vi "SwerveCalculation.vi"(6 "Rot. Point Y":dbl, 7 "Rot. Point X":dbl, 8 "Field Concentric":bool, 9 "Z":dbl(knob) scale=1.0..-1.0, 10 "Y":dbl(slide) scale=1.0..-1.0, 11 "X":dbl(slide) scale=-1.0..1.0) -> ()   [LabVIEW 2016]
uses:
  Robot Global Data.vi
panel:
  in  "Auto Controls":bool
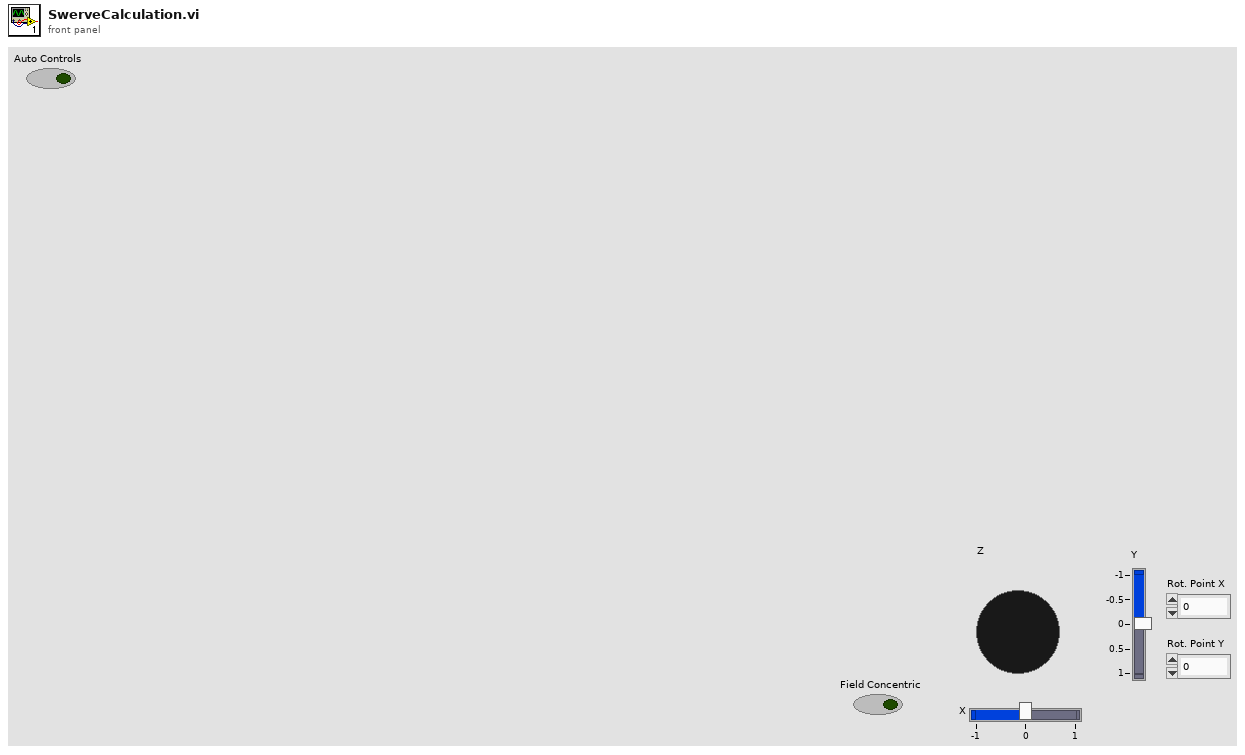
[diagram p1: front panel]
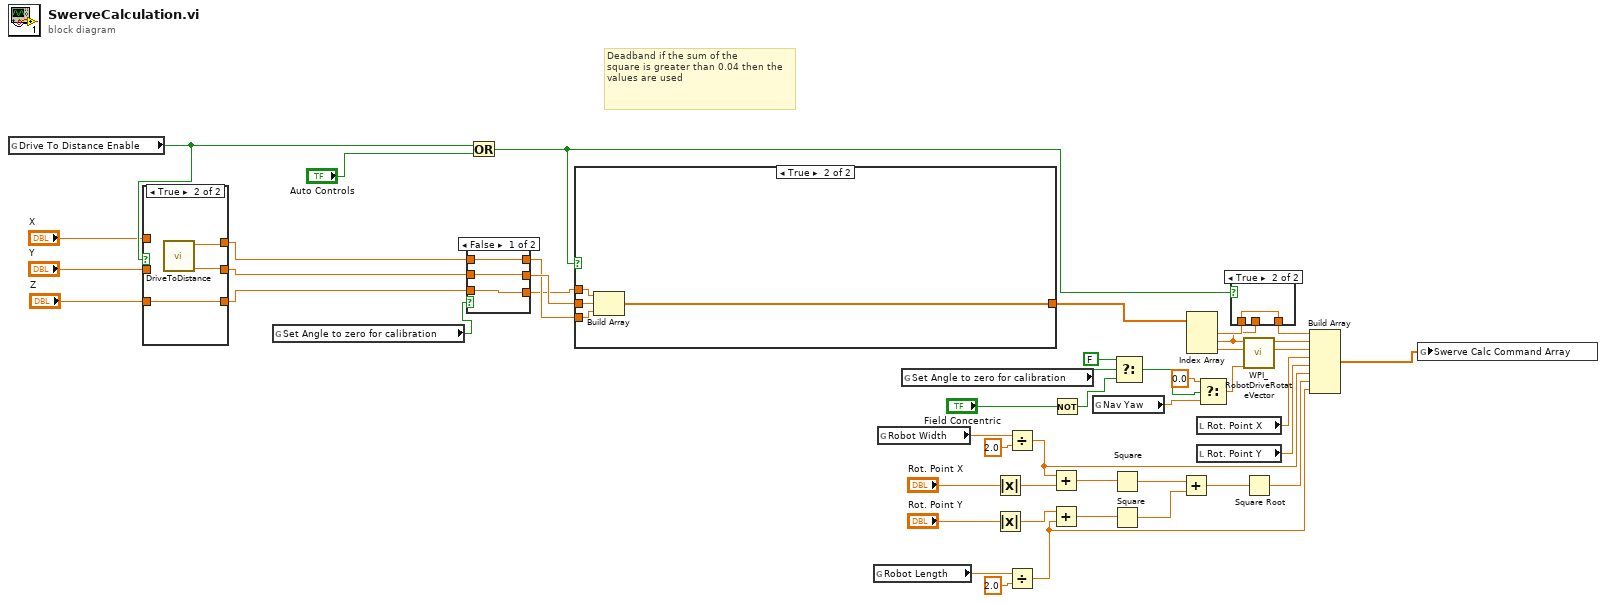
[diagram p0: block diagram]
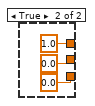
[diagram p3: hidden frame]
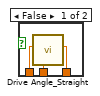
[diagram p4: hidden frame]
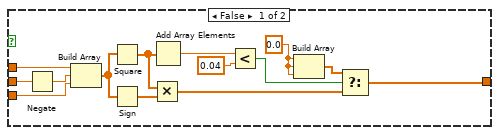
[diagram p5: hidden frame]
diagram:
  # "Deadband if the sum of the \nsquare is greater than 0.04 then the \nvalues are used"
  n1 = global read "Robot Global Data.vi" "Drive To Distance Enable"() -> (w8:bool)
  n2 = case shown="True" w8 {
    tunnel: "Z" -> [w50 w53]
    tunnel: [w50 w53] -> w6
    tunnel: "Y" -> [w49 _]
    tunnel: [w49 w51] -> w4
    tunnel: [w48 w52] -> w2
    tunnel: "X" -> [w48 _]
    frame False {
    }
    frame True {
      n3 = call "DriveToDistance.vi"() -> ("Drive Y Command"=w51:dbl, "Drive X Command"=w52:dbl)  [unwired: 10 in]
    }
  }
  n4 = global read "Robot Global Data.vi" "Set Angle to zero for calibration"() -> (w17:bool)
  n5 = case shown="False" w17 {
    tunnel: w4 -> [w56 _]
    tunnel: [w56 0.0 ("Y")] -> w20
    tunnel: w2 -> [w55 _]
    tunnel: [w55 1.0 ("X")] -> w19
    tunnel: w6 -> [w54 _]
    tunnel: [w54 0.0 ("Z")] -> w18
    frame False {
    }
    frame True {
    }
  }
  n6 = Or(x=w8, y="Auto Controls") -> (x .or. y?=w9:bool)
  n7 = case shown="True" w9 {
    tunnel: [w63 w77] -> w47
    tunnel: w19 -> [w62 w76]
    tunnel: w18 -> [w60 w75]
    tunnel: w20 -> [w61 w74]
    frame False {
      w69 = 0.0 ("element")
      n8 = Negate(x=w61) -> (-x=w65:dbl)
      n9 = Build Array(w60, w65, w62) -> (w68:dbl[])
      n10 = Square(x=w68) -> (x^2=w66:dbl[])
      n11 = Sign(1:w68) -> (0:w67:dbl[])
      n12 = Multiply(x=w66, y=w67) -> (x*y=w64:dbl[])
      n13 = Add Array Elements(numeric array=w66) -> (sum=w73:dbl)
      n14 = Less?(x=w73, y=0.04 ("x")) -> (x < y?=w71:bool)
      n15 = Build Array(w69, w69, w69) -> (w70:dbl[])
      n16 = Select(t=w70, s=w71, f=w64) -> (s? t:f=w63:dbl[])
    }
    frame True {
      n17 = Build Array(w75, w74, w76) -> (w77:dbl[])
    }
  }
  n18 = global read "Robot Global Data.vi" "Robot Length"() -> (w25:dbl)
  n19 = global read "Robot Global Data.vi" "Robot Width"() -> (w26:dbl)
  n20 = global read "Robot Global Data.vi" "Set Angle to zero for calibration"() -> (w16:bool)
  n21 = Absolute Value(x="Rot. Point X") -> (abs(x)=w42:dbl)
  n22 = Absolute Value(x="Rot. Point Y") -> (abs(x)=w40:dbl)
  n23 = Divide(x=w26, y=2.0) -> (x/y=w31:dbl)
  n24 = Divide(x=w25, y=2.0) -> (x/y=w33:dbl)
  n25 = Add(x=w31, y=w42) -> (x+y=w41:dbl)
  n26 = Add(x=w40, y=w33) -> (x+y=w39:dbl)
  n27 = Not(x="Field Concentric") -> (.not. x?=w15:bool)
  n28 = global read "Robot Global Data.vi" "Nav Yaw"() -> (w44:dbl)
  n29 = Square(x=w41) -> (x^2=w37:dbl)
  n30 = Square(x=w39) -> (x^2=w38:dbl)
  n31 = Select(t=FALSE, s=w16, f=w15) -> (s? t:f=w14:bool)
  n32 = Add(x=w37, y=w38) -> (x+y=w36:dbl)
  n33 = Index Array(array=w47) -> (element #1=w22:dbl, element #2=w11:dbl, element #3=w12:dbl)  [unwired: 3 in]
  n34 = local read "Rot. Point X"() -> (w30:dbl)
  n35 = local read "Rot. Point Y"() -> (w29:dbl)
  n36 = Select(t=0.0, s=w14, f=w44) -> (s? t:f=w43:dbl)
  n37 = case shown="True" w9 {
    tunnel: w22 -> [w80 w81]
    tunnel: [w79 w81] -> w21
    tunnel: w11 -> [w78 _]
    frame False {
      n38 = call "Drive Angle_Straight.vi"("y input"=w78, "Z axis in"=w80) -> ("Z out"=w79:dbl)  [unwired: 9 in]
    }
    frame True {
    }
  }
  n39 = call <vilib>:"WPI_RobotDriveRotateVector.vi"("Angle"=w43, "X"=w12, "Y"=w11) -> ("X'"=w28:dbl, "Y'"=w27:dbl)  [unwired: 7 out]
  n40 = Square Root(x=w36) -> (sqrt(x)=w32:dbl)
  n41 = Build Array(w21, w27, w28, w30, w29, w31, w32, w33) -> (w1:dbl[])
  n42 = global write "Robot Global Data.vi" "Swerve Calc Command Array"(w1) -> ()
